vi "REMOND Studio_DO Water Q.vi"() -> ()   [LabVIEW 2021]
uses:
  FSM_States.ctl
  Global_Message.ctl
  <vilib>/Modbus/master/Modbus Master.lvclass
  <vilib>/Utility/error.llb/DialogType.ctl
  Global_flags.vi
  <vilib>/Modbus/master/Create Master Instance (Serial).vi
panel:
  in  "Measure Mode":u16(ring)=1 items=["[%]", "[mg/L]"]
  out "Tiempo Actual":string
  out "ADC":u16
  in  "Confirm Slope":bool
  in  "Confirm Zero":bool
  in  "Start Calib":bool
  out "Warning :":string
  out "Current Out Val :":sgl format="%#.3f"
  out "Temperature [°C]:":sgl format="%#.1f °C"
  out "Measurement [%  ; mg/L]:":sgl format="%#.2f mg/L"
  in  "Exit":bool
  in  "Restore Default":bool
  in  "Adquire / Stop":bool
  in  "SetBaudRate":bool
  in  "BaudRate (9600)":u16(ring)=2 items=["2400", "4800", "9600", "19200", "38400"]
  in  "Addr Set":u16=1 min=1 max=255 step=1
  in  "SetAddress":bool
  in  "D.S":u16(ring)=1 items=["0.5s", "1s", "1.5s", "2.0s", "2.5s", "3.0s", "3.5s", "4.0s", "4.5s", "5.0s"]
  in  "BaudRate (9600)":u32=9600 min=2400 max=38400 step=1
  in  "Address":u8=1 min=1 step=1
  in  "Open/Close COM":bool
  in  "COM":refnum<visa-resource-name>
  out "Consumer Shutdown?":bool
  # "Calibracion:"
  # "ADC :"
  # "Start CALIB --- >>> STOP ADQRUIING , DISble and gray out Measur and SHow ADC"
  # "Evento de filtrado Calib Slope Optional !!"
  # "Disable and gray out Measurements (Prop Node) while calibrating"
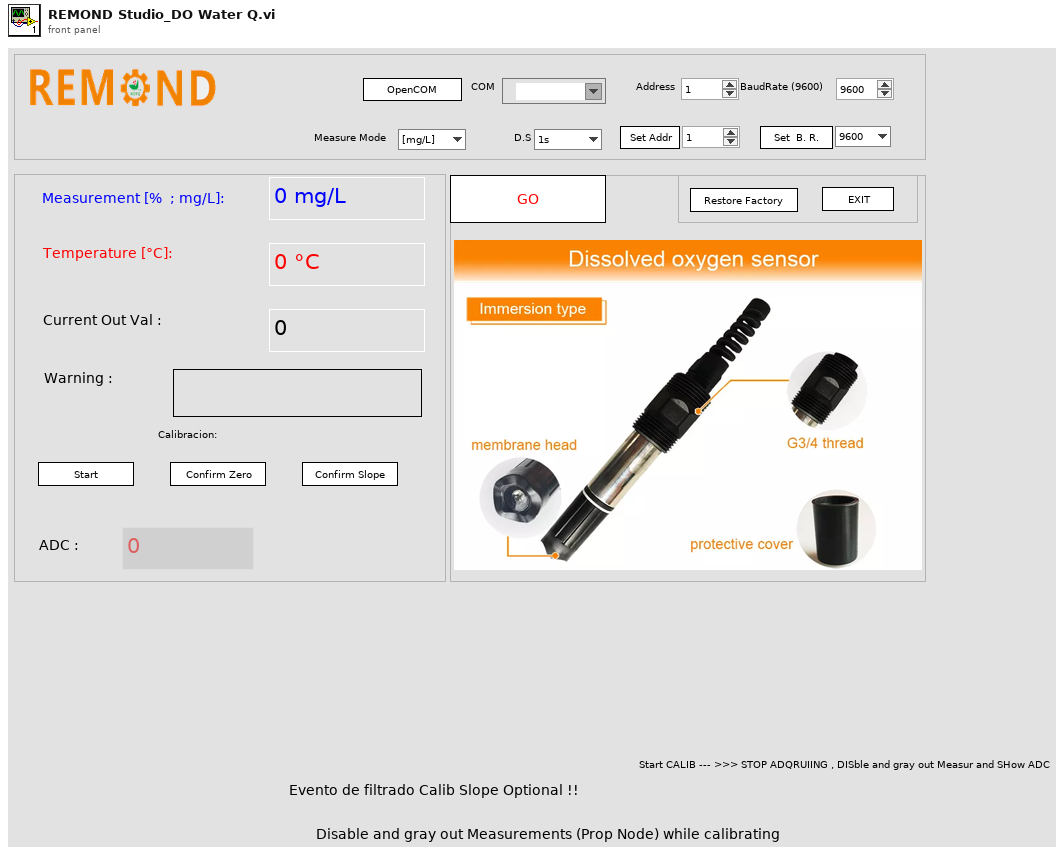
[diagram p1: front panel]
types:
  T1 = typedef "Global_Message.ctl" = cluster{"Consumer State":T2, "User Msg":string, "error in (no error)":errorcluster, "User Msg 2":string}
  T2 = typedef "FSM_States.ctl" = enum16{"Set Measure Mode", "Initialize", "Open COM Port", "Adquire Data", "Set Address", "Set BaudRate", "Restore Factory", "Pre-Set Zero", "Pre-Set K=1", "Pre-Set Slope", "Confirm Zero", "Confirm Slope", "Confirm EC", "Close COM Port", "Exit App", "Stop Data", "Calibrate sensor"}
  T3 = enum8{"Enabled", "Disabled", "Disabled and Grayed Out"}
  T4 = typedef "DialogType.ctl" = u16
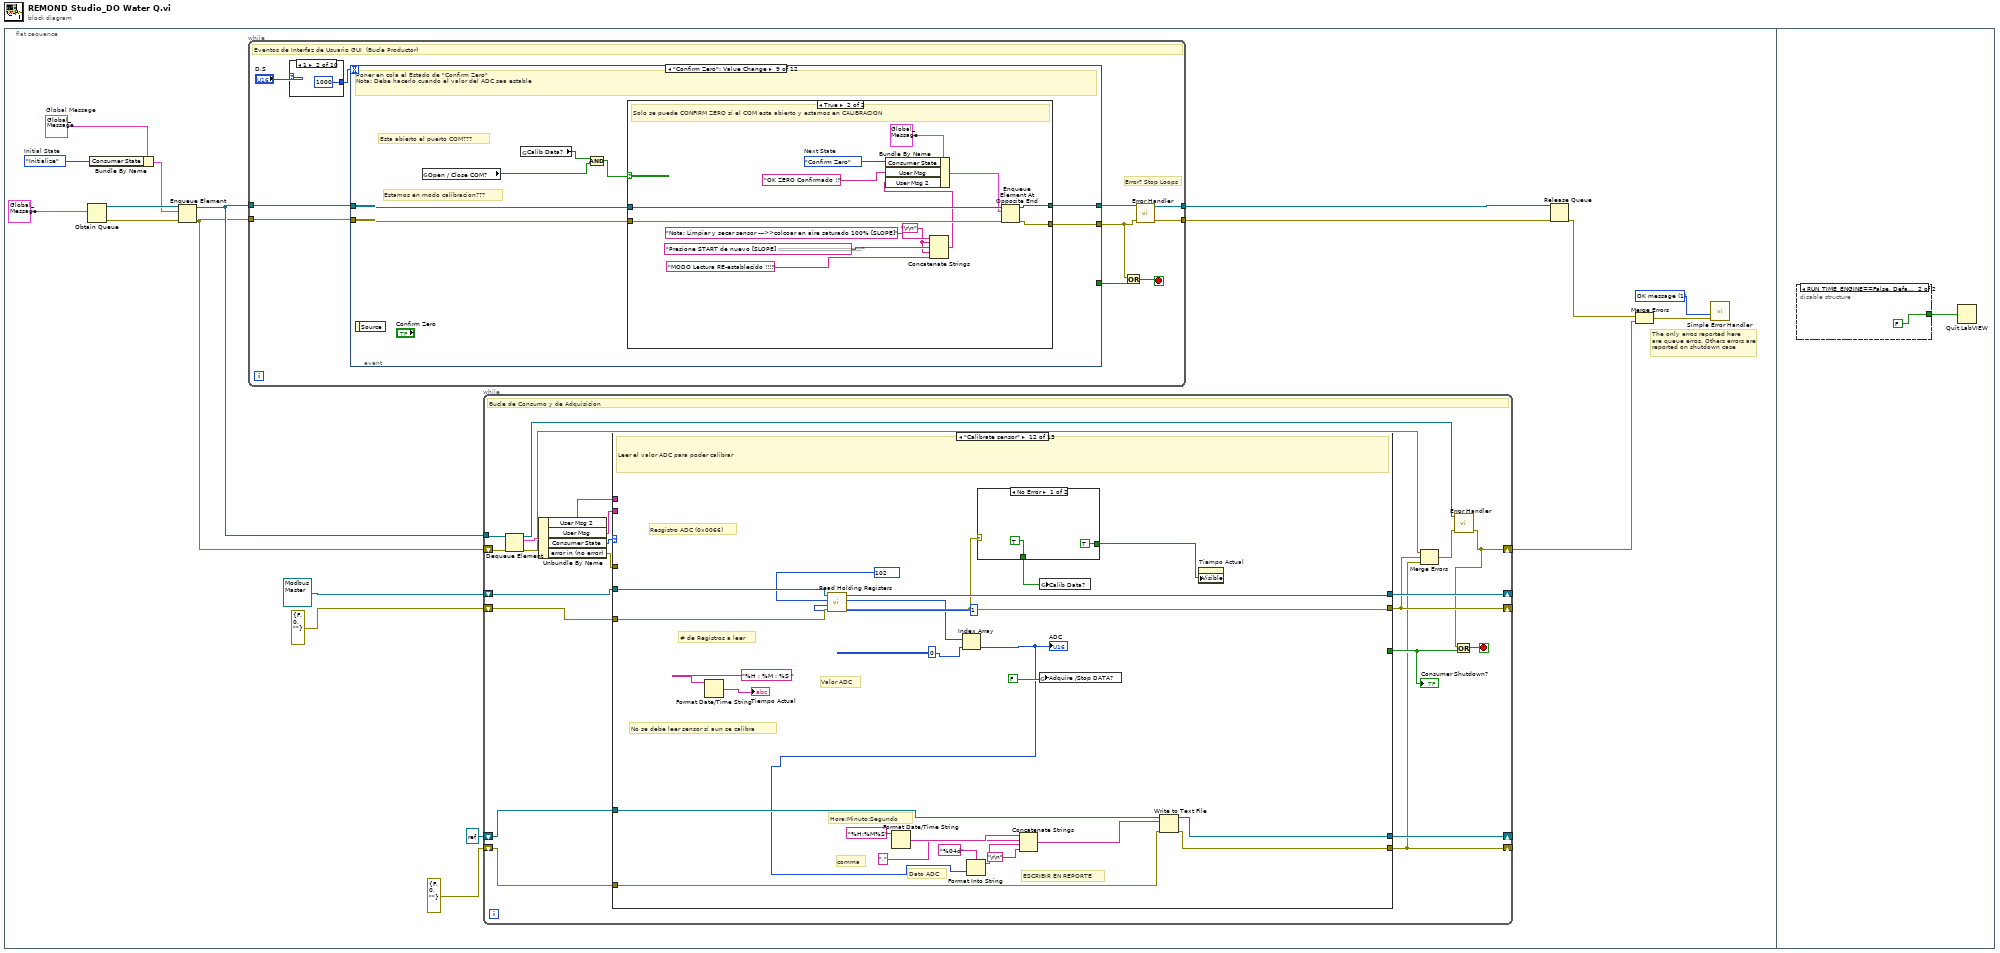
[diagram p0: block diagram]
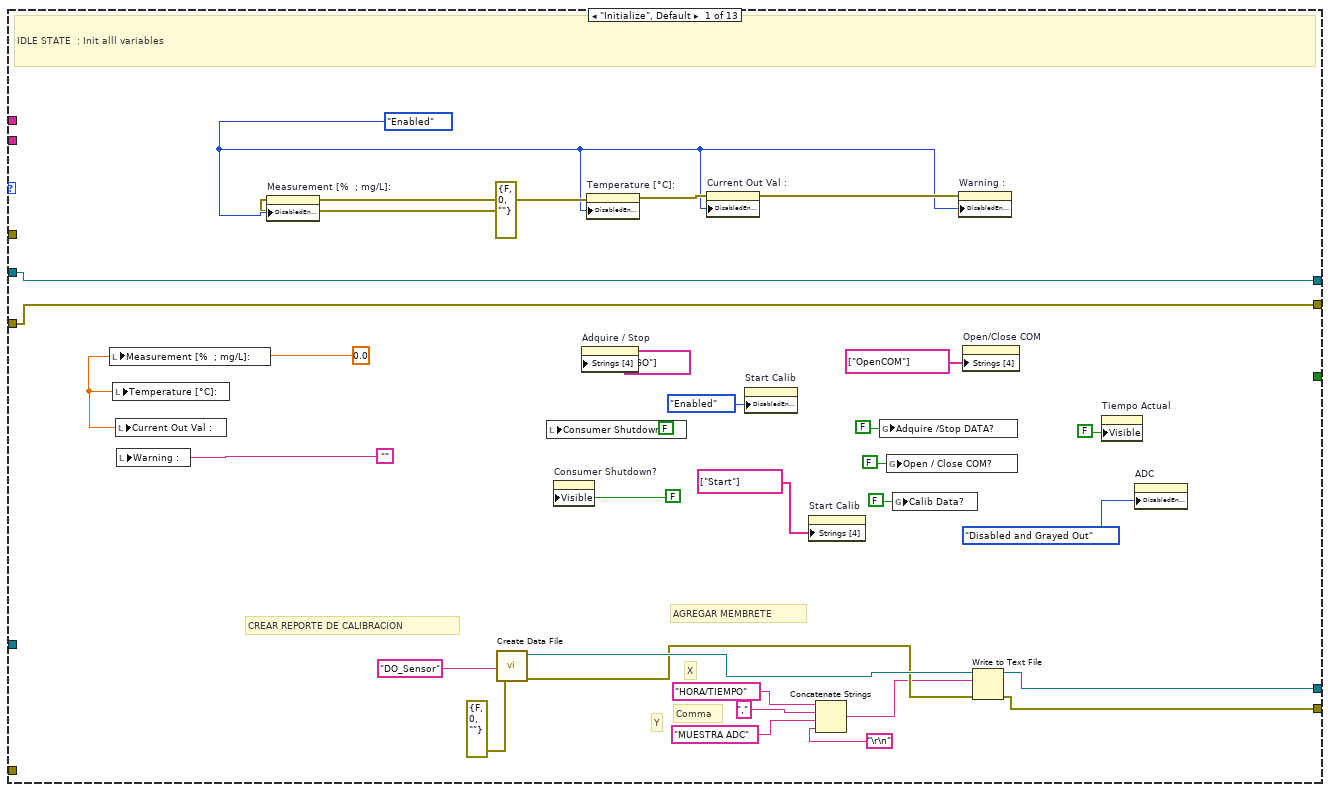
[diagram p2: hidden frame]
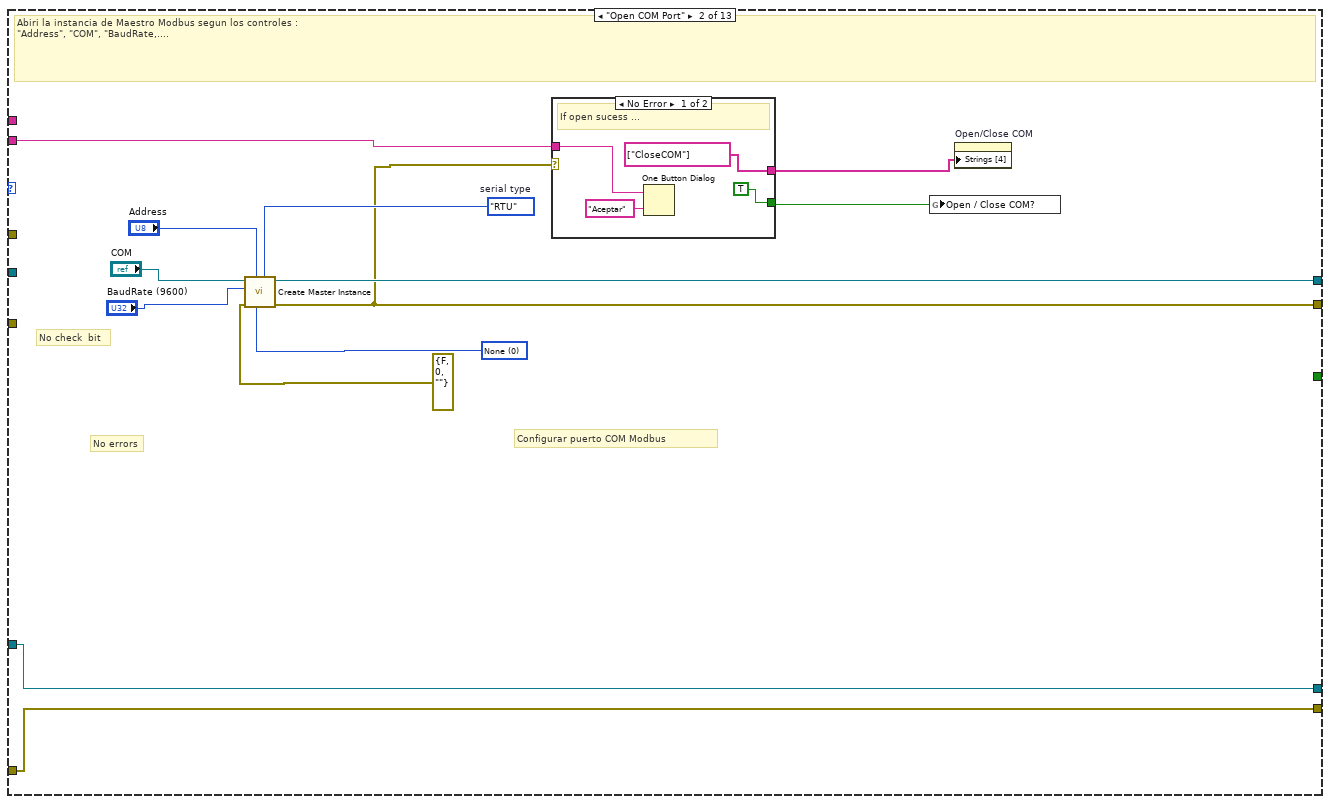
[diagram p3: hidden frame]
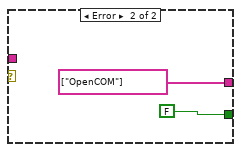
[diagram p4: hidden frame]
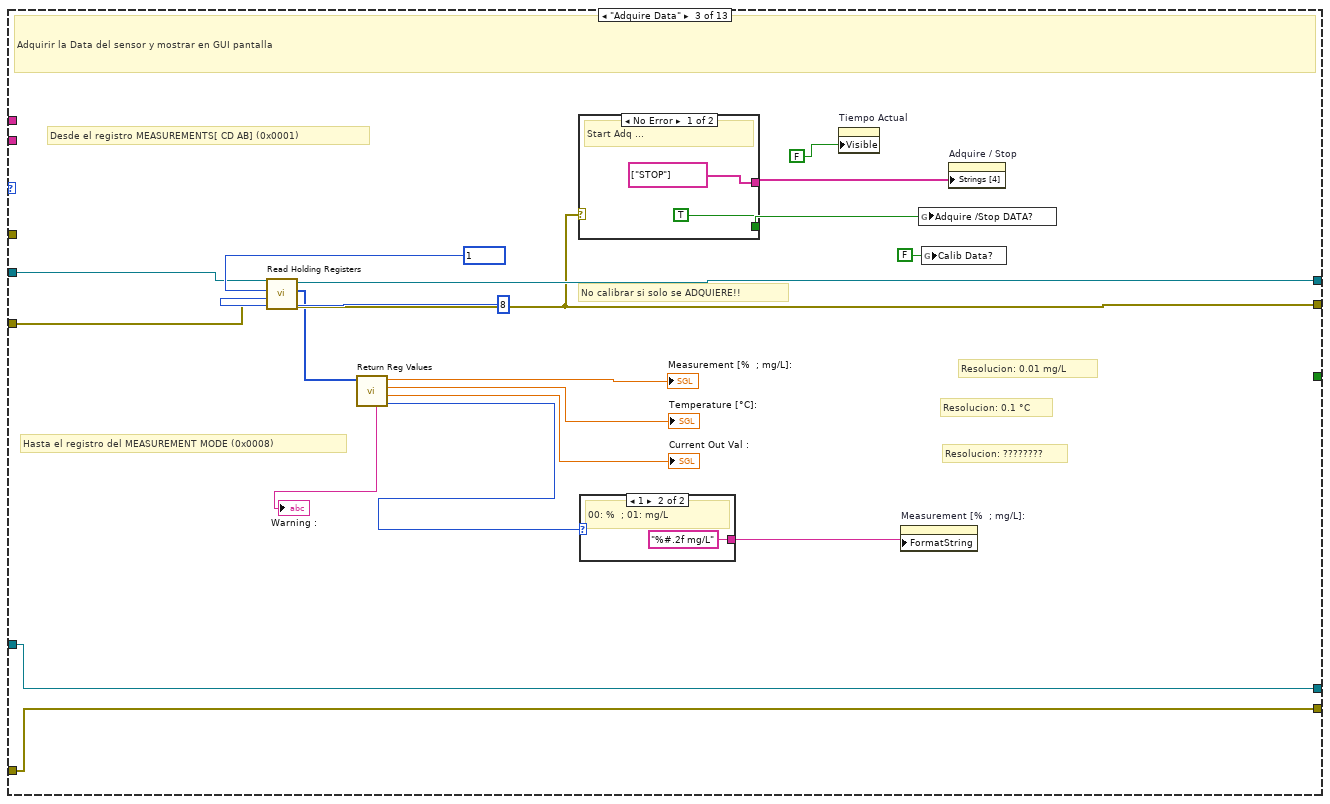
[diagram p5: hidden frame]
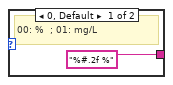
[diagram p6: hidden frame]
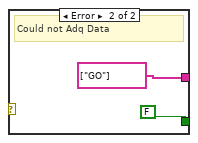
[diagram p7: hidden frame]
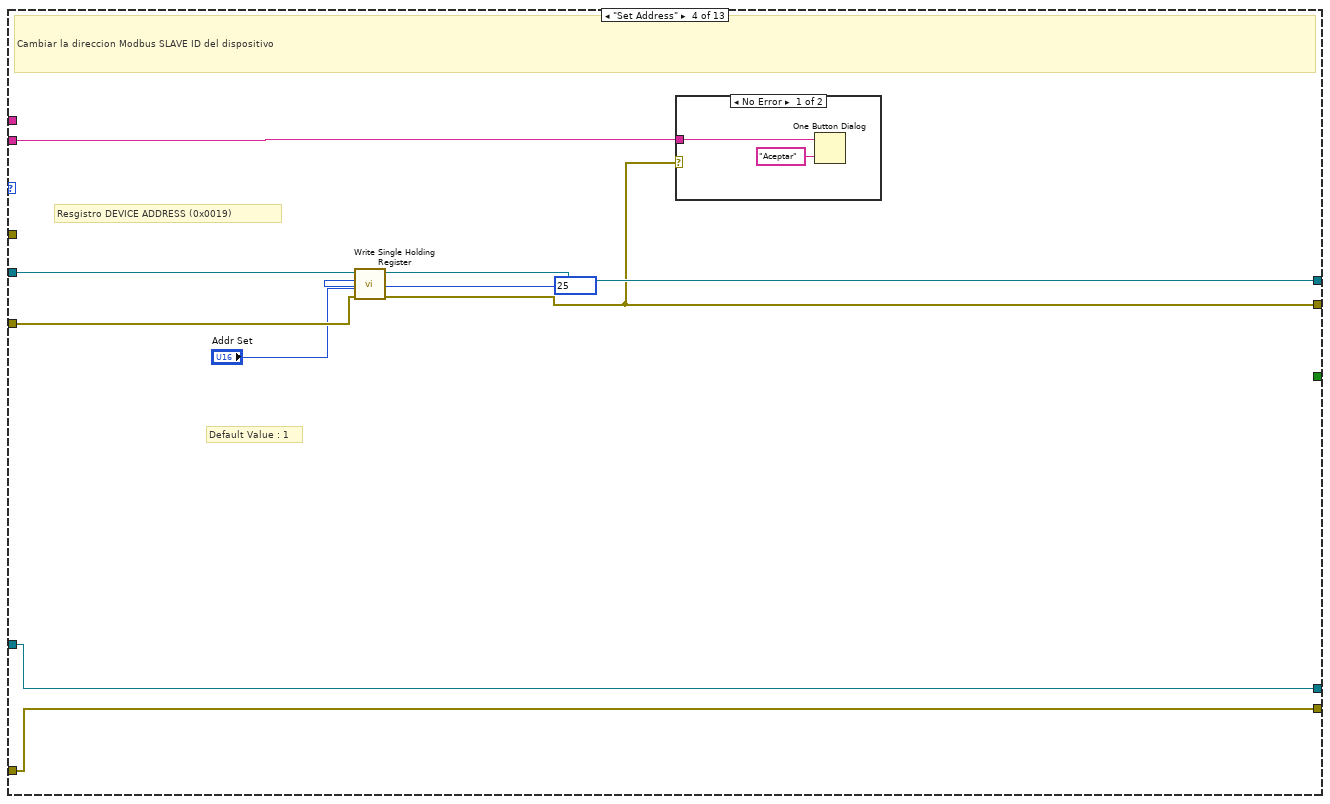
[diagram p8: hidden frame]
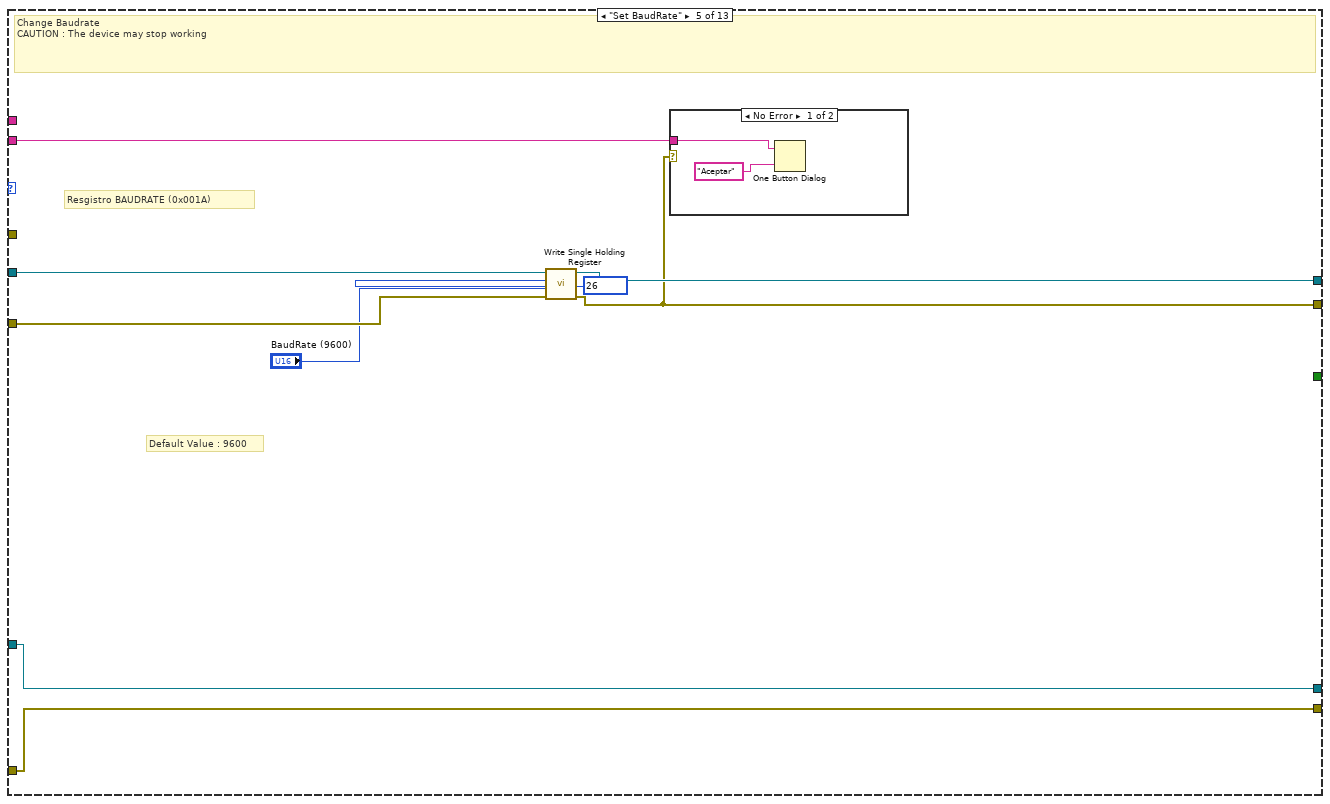
[diagram p10: hidden frame]
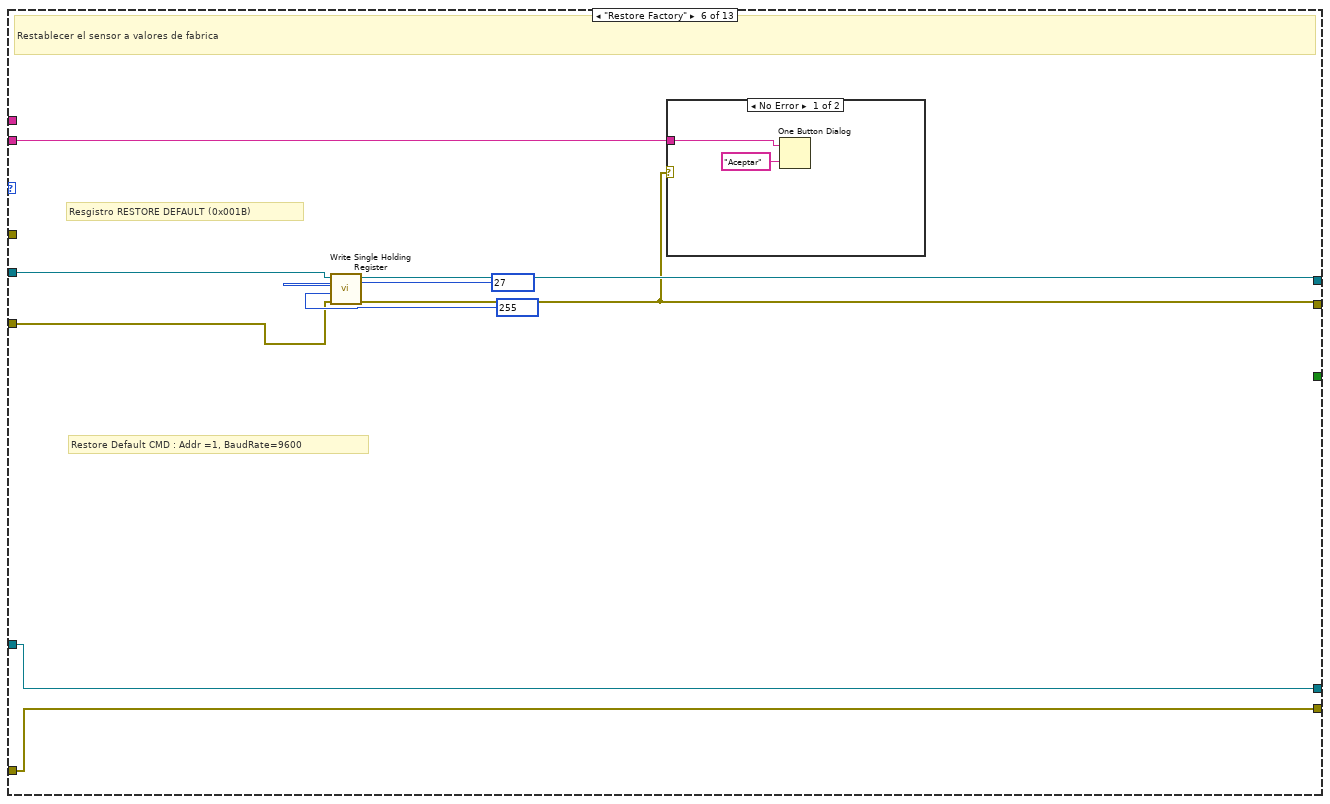
[diagram p12: hidden frame]
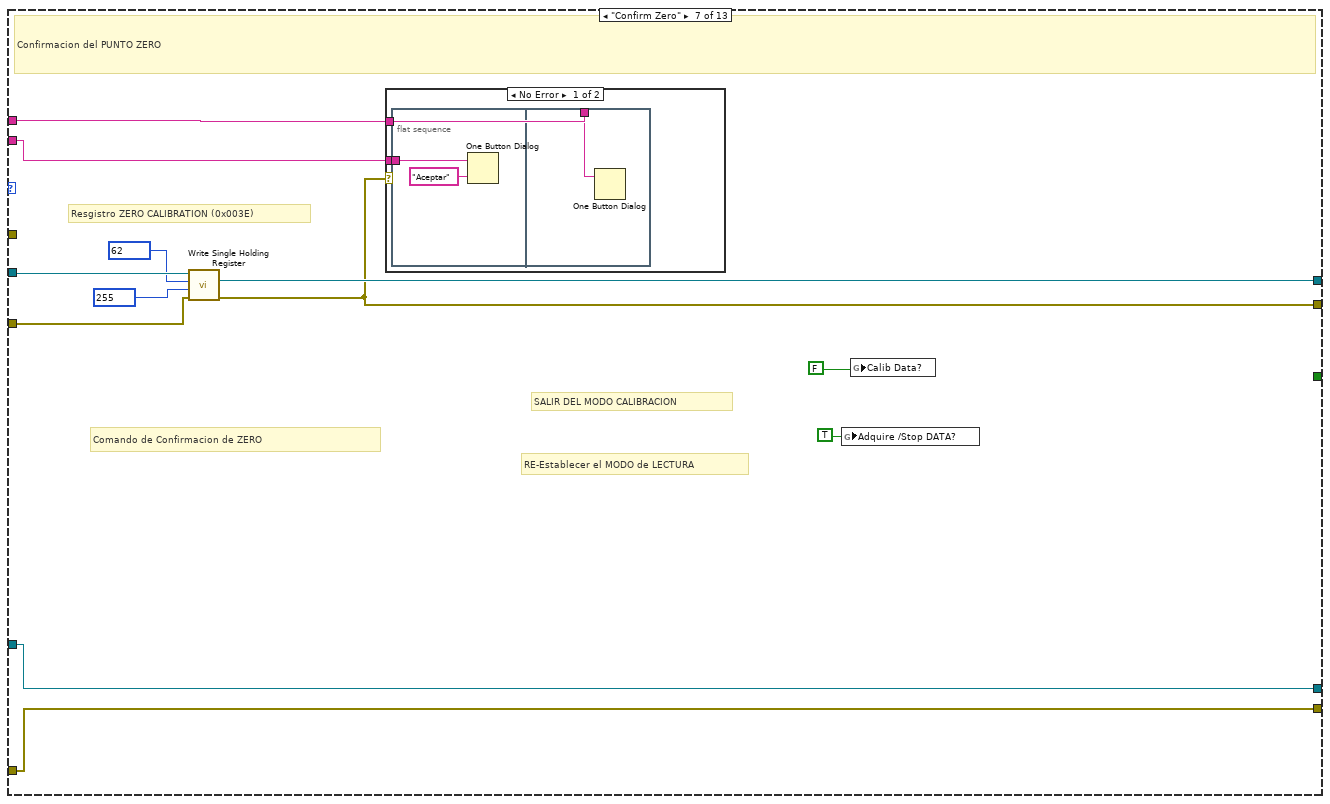
[diagram p14: hidden frame]
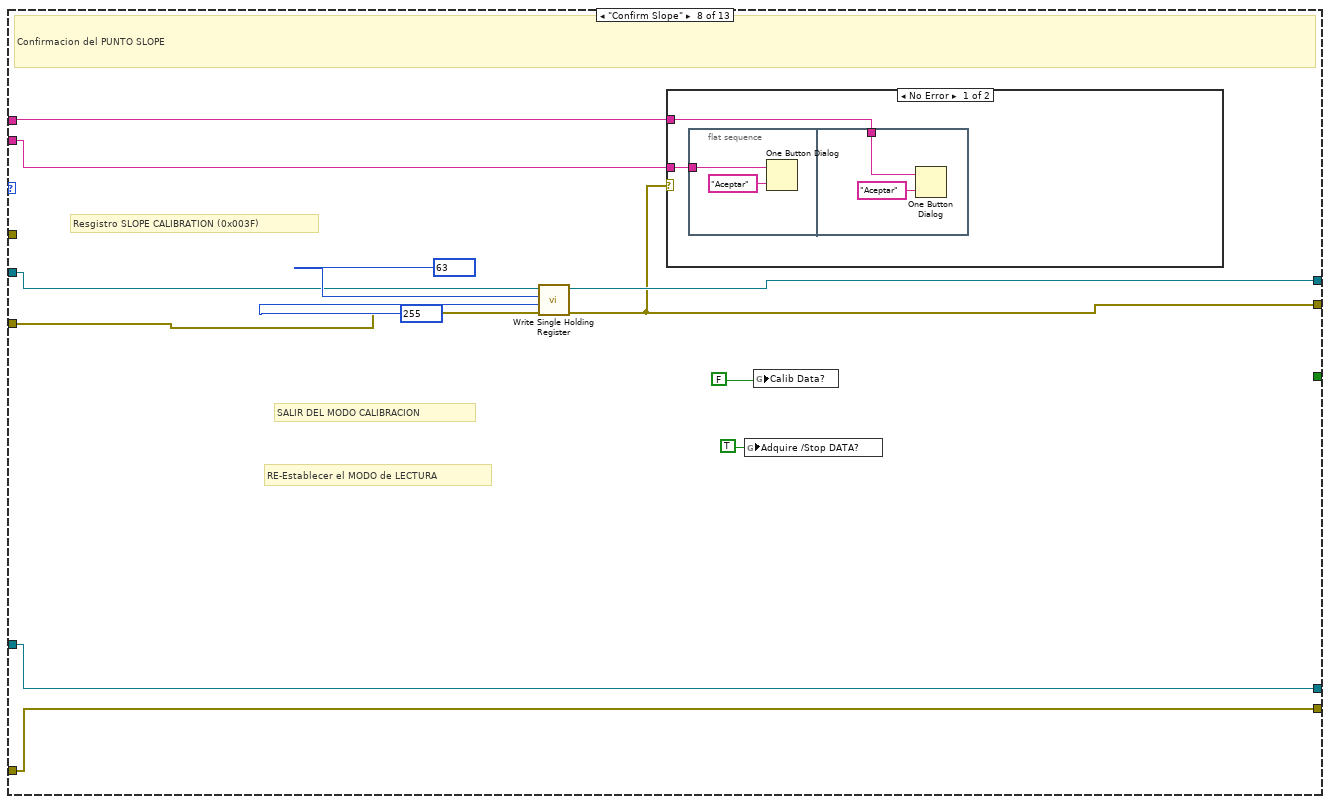
[diagram p16: hidden frame]
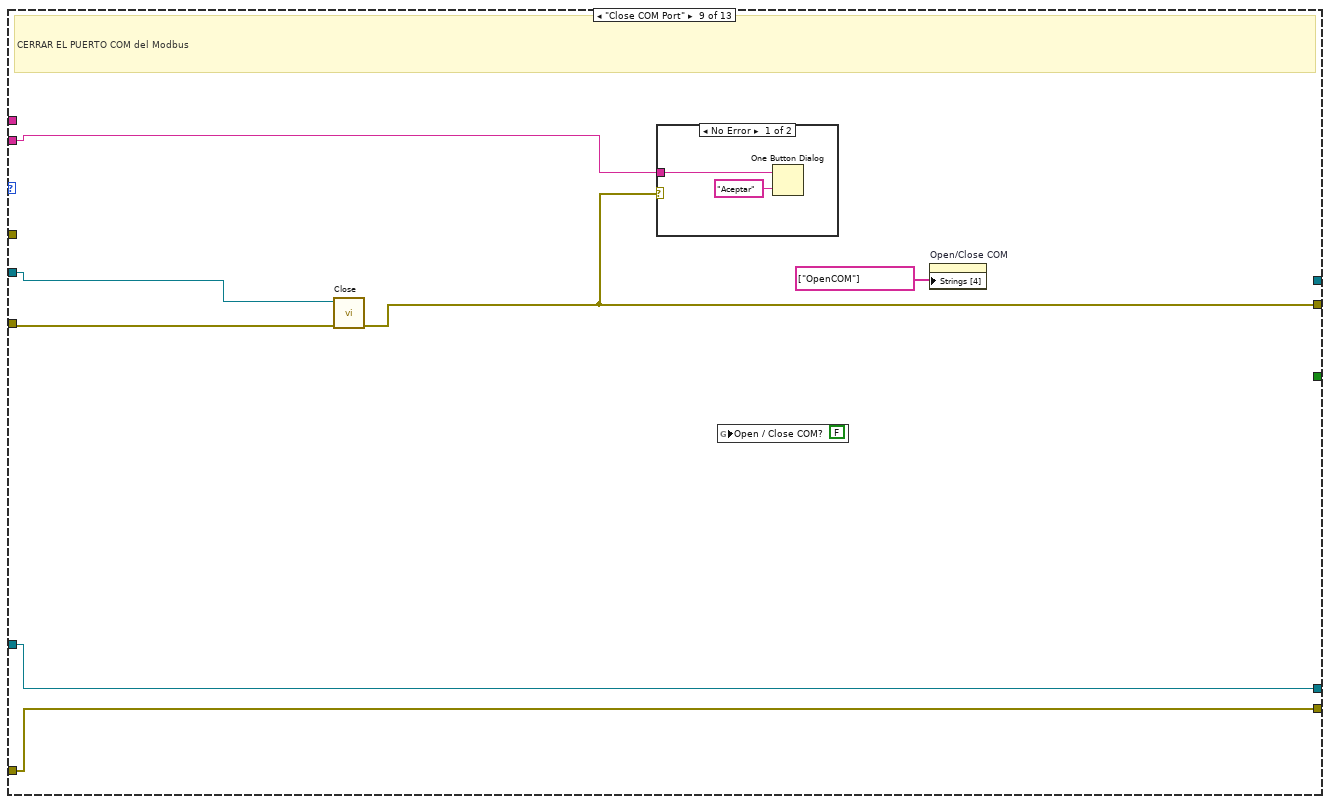
[diagram p18: hidden frame]
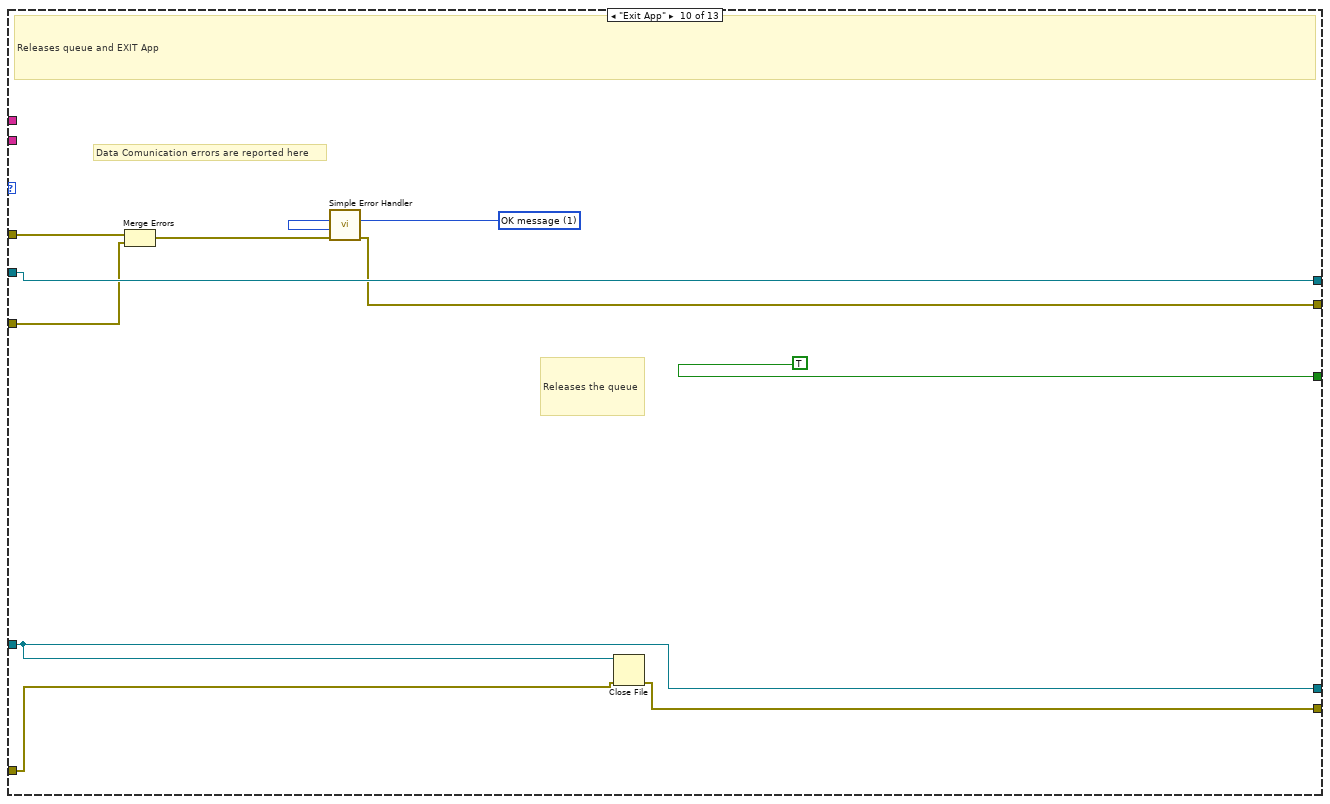
[diagram p20: hidden frame]
diagram:
  n1 = flat-sequence {
    frame #0 {
      w5 = T4 1 items=["no dialog", "OK message", "continue or stop message", "OK message + warnings", "continue/stop + warnings"] ("type of dialog (OK msg:1)")
      w15 = T1 {"Consumer State"=enum."Open COM Port", "User Msg"="", "error in (no error)"={"status"=FALSE, "code"=0, "source"=""}, "User Msg 2"=""}  # Global Message
      w14 = FSM_States."Initialize"  # Initial State
      # "The only erros reported here\nare queue erros. Others errors are\nreported on shutdown case"
      n2 = Obtain Queue(element data type=T1 {"Consumer State"=enum."Open COM Port", "User Msg"="", "error in (no error)"={"status"=FALSE, "code"=0, "source"=""}, "User Msg 2"=""} ("Global Message")) -> (queue out=w17:refnum<queue>, error out=w16:errorcluster)  [unwired: 4 in, 1 out]
      n3 = Bundle By Name(cluster=w15, "Consumer State"=w14) -> (w13:T1)
      n4 = Enqueue Element(queue=w17, element=w13, error in (no error)=w16) -> (queue out=w12:refnum<queue>, error out=w11:errorcluster)  [unwired: 1 in, 1 out]
      n5 = while {
        tunnel: w12 -> [w264]
        tunnel: w11 -> [w263]
        tunnel: [w259] -> w8
        tunnel: [w258] -> w7
        stop <- w255 stop-if-true
        # "Error? Stop Loops"
        # "Eventos de Interfaz de Usuario GUI  (Bucle Productor)"
        n6 = case shown="1" "D.S" {
          tunnel: [500 1000 1500 2000 2500 3000 3500 4000 4500 5000] -> w262
          frame 0, Default {
          }
          frame 1 {
          }
          frame 2 {
          }
          frame 3 {
          }
          frame 4 {
          }
          frame 5 {
          }
          frame 6 {
          }
          frame 7 {
          }
          frame 8 {
          }
          frame 9 {
          }
        }
        n7 = event shown="[8] \"Confirm Zero\": Value Change" {
          selector: _ -> [_ _ _ _ _ _ _ _ _ _ _ _]
          dyn-events: _ -> [_ _ _ _ _ _ _ _ _ _ _ _]
          timeout: w262 -> [_ _ _ _ _ _ _ _ _ _ _ _]
          tunnel: w264 -> [w285 w307 w322 w346 w383 w403 w423 w443 w485 w512 w537 w555]
          tunnel: w263 -> [w284 w306 w321 w345 w381 w401 w421 w441 w483 w510 w535 w554]
          tunnel: [w283 w305 w320 w344 w382 w402 w422 w442 w484 w511 w536 w555] -> w260
          tunnel: [w282 w304 w319 w343 w380 w400 w420 w440 w482 w509 w534 w554] -> w256
          tunnel: [w281 _ _ _ _ _ _ _ _ _ w532 _] -> w257
          event Timeout {
            # "Para ADQUIRIR DATOS, se debe ABRIR el PUERTO COM"
            # "Poner en cola el estado de \"ADQUIRE DATA\" de forma automatica cada 1000 mseg\n\nNOTA: Solo funcionara si el puerto COM esta abierto"
            n8 = event-data() -> ()  [unwired: 1 in, 1 out]
            n9 = global read "Global_flags.vi" "Adquire /Stop DATA?"() -> (w275:bool)
            n10 = case shown="True" w275 {
              frame False {
              }
              frame True {
                w286 = T3."Enabled" ("Disabled")
                # "Si se vuelve a adquirir, mostrar los controles"
                n11 = property on="Measurement [%  ; mg/L]:" class="DigNum (strict)"("DisabledEnum"=w286) -> ()  [unwired: 2 in, 2 out]
                n12 = property on="Temperature [°C]:" class="DigNum (strict)"("DisabledEnum"=w286) -> ()  [unwired: 2 in, 2 out]
                n13 = property on="Current Out Val :" class="DigNum (strict)"("DisabledEnum"=w286) -> ()  [unwired: 2 in, 2 out]
                n14 = property on="ADC" class="DigNum (strict)"("DisabledEnum"=T3."Disabled and Grayed Out" ("Disabled")) -> ()  [unwired: 2 in, 2 out]
                n15 = property on="Warning :" class="Str"("DisabledEnum"=w286) -> ()  [unwired: 2 in, 2 out]
                n16 = property on="Start Calib" class="Bool"("DisabledEnum"=w286) -> ()  [unwired: 2 in, 2 out]
              }
            }
            n17 = global read "Global_flags.vi" "Calib Data?"() -> (w280:bool)
            n18 = global read "Global_flags.vi" "Open / Close COM?"() -> (w278:bool)
            n19 = Build Array(w275, w280) -> (w279:bool[])
            n20 = And(x=w279, y=w278) -> (x .and. y?=w277:bool[])
            n21 = Boolean Array To Number(Boolean array=w277) -> (number=w276:u32)
            n22 = case shown="2" w276 {
              tunnel: [w289 w294 w300] -> w283
              tunnel: [w288 w293 w298] -> w282
              tunnel: w285 -> [w289 w291 w301]
              tunnel: w284 -> [w288 w290 w299]
              frame 0, Default {
                # "Caso contrario, Bypass"
              }
              frame 1 {
                w292 = FSM_States."Adquire Data"  # Next State
                # "Si Adq/Stop ==True entonces ADQUIRIR"
                n23 = Bundle By Name(cluster=T1 {"Consumer State"=enum."Open COM Port", "User Msg"="", "error in (no error)"={"status"=FALSE, "code"=0, "source"=""}, "User Msg 2"=""} ("Global Message"), "Consumer State"=w292) -> (w295:T1)
                n24 = Enqueue Element(queue=w291, element=w295, error in (no error)=w290) -> (queue out=w294:refnum<queue>, error out=w293:errorcluster)  [unwired: 1 in, 1 out]
              }
              frame 2 {
                w303 = FSM_States."Calibrate sensor"  # Next State
                # "Si Calib Data? == True entonces calibrar sensor"
                n25 = Bundle By Name(cluster=T1 {"Consumer State"=enum."Open COM Port", "User Msg"="", "error in (no error)"={"status"=FALSE, "code"=0, "source"=""}, "User Msg 2"=""} ("Global Message"), "Consumer State"=w303) -> (w297:T1)
                n26 = Enqueue Element(queue=w301, element=w297, error in (no error)=w299) -> (queue out=w300:refnum<queue>, error out=w298:errorcluster)  [unwired: 1 in, 1 out]
              }
            }
            n27 = local read "Consumer Shutdown?"() -> (w281:bool)
          }
          event "Open/Close COM": Value Change {
            w313 = FSM_States."Close COM Port"  # Next State
            w314 = FSM_States."Open COM Port"  # Next State
            # "Poner en cola en estado de apertura de puerto COM Modbus"
            n28 = event-data() -> ()  [unwired: 1 in, 1 out]
            n29 = global read "Global_flags.vi" "Open / Close COM?"() -> (w311:bool)
            n30 = Select(t="Puerto COM cerrado !", s=w311, f="Puerto COM abierto !" ("User Msg")) -> (s? t:f=w310:string)
            n31 = Select(t=w313, s=w311, f=w314) -> (s? t:f=w316:T2)
            n32 = Bundle By Name(cluster=T1 {"Consumer State"=enum."Open COM Port", "User Msg"="", "error in (no error)"={"status"=FALSE, "code"=0, "source"=""}, "User Msg 2"=""} ("Global Message"), "Consumer State"=w316, "User Msg"=w310) -> (w309:T1)
            n33 = Enqueue Element(queue=w307, element=w309, error in (no error)=w306) -> (queue out=w305:refnum<queue>, error out=w304:errorcluster)  [unwired: 1 in, 1 out]
          }
          event "Measure Mode": Value Change {
            # "Esta abierto el puerto COM???"
            # "Poner en cola en estado de MODO\nNOTA: Solo funcionara si el COM esta abierto"
            n34 = event-data() -> ()  [unwired: 1 in, 4 out]
            n35 = global read "Global_flags.vi" "Open / Close COM?"() -> (w318:bool)
            n36 = case shown="True" w318 {
              tunnel: w322 -> [w324 w335]
              tunnel: w321 -> [w323 w334]
              tunnel: [w324 w333] -> w320
              tunnel: [w323 w332] -> w319
              tunnel: "Measure Mode" -> [_ w331]
              frame False {
                # "Solo se puede SET MEASU MODE si el COM esta abierto"
                n37 = Concatenate Strings("Para cambiar MEASURE MODE::::::" ("message"), "\r\n", "Debe ABRIR Puerto COM !!!" ("string")) -> (w329:string)
                n38 = One Button Dialog(message=w329, button name ("OK")="Aceptar") -> ()  [unwired: 1 out]
              }
              frame True {
                w338 = FSM_States."Set Measure Mode"  # Next State
                # "Solo se puede SET MEASU MODE si el COM esta abierto"
                n39 = case shown="0, Default" w331 {
                  tunnel: ["%" "mg/L"] -> w330
                  frame 0, Default {
                  }
                  frame 1 {
                  }
                }
                n40 = Bundle By Name(cluster=T1 {"Consumer State"=enum."Open COM Port", "User Msg"="", "error in (no error)"={"status"=FALSE, "code"=0, "source"=""}, "User Msg 2"=""} ("Global Message"), "Consumer State"=w338, "User Msg"="OK Measure Mode Changed!!! !!", "User Msg 2"=w330) -> (w336:T1)
                n41 = Enqueue Element(queue=w335, element=w336, error in (no error)=w334) -> (queue out=w333:refnum<queue>, error out=w332:errorcluster)  [unwired: 1 in, 1 out]
              }
            }
          }
          event "Adquire / Stop": Value Change {
            # "Esta abierto el puerto COM???"
            # "Ya se esta adquiriendo???"
            # "Poner en cola en estado de adquisicion de muestras\nNOTA: Solo funcionara si el COM esta abierto"
            n42 = event-data() -> ()  [unwired: 1 in, 1 out]
            n43 = global read "Global_flags.vi" "Adquire /Stop DATA?"() -> (w347:bool)
            n44 = global read "Global_flags.vi" "Open / Close COM?"() -> (w342:bool)
            n45 = case shown="True" w342 {
              tunnel: w347 -> [_ w364]
              tunnel: w346 -> [w354 w363]
              tunnel: w345 -> [w353 w362]
              tunnel: [w354 w361] -> w344
              tunnel: [w353 w360] -> w343
              frame False {
                # "Solo se puede ADQUIRIR si el COM esta abierto"
                n46 = Concatenate Strings("Para ADQUIRI muestras::::::" ("message"), "\r\n", "Debe ABRIR Puerto COM !!!" ("string")) -> (w348:string)
                n47 = One Button Dialog(message=w348, button name ("OK")="Aceptar") -> ()  [unwired: 1 out]
              }
              frame True {
                w355 = T3."Enabled" ("Disabled")
                w356 = errorcluster {"status"=FALSE, "code"=0, "source"=""} ("error in (no error)")
                # "Solo se puede ADQUIRIR si el COM esta abierto"
                n48 = property on="Measurement [%  ; mg/L]:" class="DigNum (strict)"(error in=w356, "DisabledEnum"=w355) -> (error out=w359:errorcluster)  [unwired: 1 in, 1 out]
                n49 = property on="Start Calib" class="Bool"(error in=w356, "DisabledEnum"=w355) -> ()  [unwired: 1 in, 2 out]
                n50 = case shown="True" w364 {
                  tunnel: [w369 w375] -> w361
                  tunnel: [w368 w374] -> w360
                  tunnel: w363 -> [w366 w373]
                  tunnel: w362 -> [w365 w372]
                  frame False {
                    w367 = FSM_States."Adquire Data"  # Next State
                    # "Si no se ha iniciado la adquisicion  encolar ADQUIRIR"
                    n51 = Bundle By Name(cluster=T1 {"Consumer State"=enum."Open COM Port", "User Msg"="", "error in (no error)"={"status"=FALSE, "code"=0, "source"=""}, "User Msg 2"=""} ("Global Message"), "Consumer State"=w367) -> (w370:T1)
                    n52 = Enqueue Element(queue=w366, element=w370, error in (no error)=w365) -> (queue out=w369:refnum<queue>, error out=w368:errorcluster)  [unwired: 1 in, 1 out]
                  }
                  frame True {
                    w376 = FSM_States."Stop Data"  # Next State
                    # "Si ya se estaba adquiriendo, DETENER la toma de data"
                    n53 = Bundle By Name(cluster=T1 {"Consumer State"=enum."Open COM Port", "User Msg"="", "error in (no error)"={"status"=FALSE, "code"=0, "source"=""}, "User Msg 2"=""} ("Global Message"), "Consumer State"=w376) -> (w377:T1)
                    n54 = Enqueue Element(queue=w373, element=w377, error in (no error)=w372) -> (queue out=w375:refnum<queue>, error out=w374:errorcluster)  [unwired: 1 in, 1 out]
                  }
                }
                n55 = property on="Temperature [°C]:" class="DigNum (strict)"(error in=w359, "DisabledEnum"=w355) -> (error out=w358:errorcluster)  [unwired: 1 in, 1 out]
                n56 = property on="Current Out Val :" class="DigNum (strict)"(error in=w358, "DisabledEnum"=w355) -> (error out=w357:errorcluster)  [unwired: 1 in, 1 out]
                n57 = property on="Warning :" class="Str"(error in=w357, "DisabledEnum"=w355) -> ()  [unwired: 1 in, 2 out]
              }
            }
          }
          event "SetAddress": Value Change {
            # "Esta abierto el puerto COM???"
            # "Poner en cola el Estado de Set Address\nNOTA: Solo funcionara si el COM esta abierto"
            n58 = event-data() -> ()  [unwired: 1 in, 1 out]
            n59 = global read "Global_flags.vi" "Open / Close COM?"() -> (w379:bool)
            n60 = case shown="False" w379 {
              tunnel: w383 -> [w390 w396]
              tunnel: [w390 w395] -> w382
              tunnel: w381 -> [w389 w394]
              tunnel: [w389 w393] -> w380
              frame False {
                # "Solo se puede SetAddr si el COM esta abierto"
                n61 = Concatenate Strings("Para cambiar SLAVE ID::::::" ("message"), "\r\n", "Debe ABRIR Puerto COM !!!" ("string")) -> (w388:string)
                n62 = One Button Dialog(message=w388, button name ("OK")="Aceptar") -> ()  [unwired: 1 out]
              }
              frame True {
                w397 = FSM_States."Set Address"  # Next State
                # "Solo se puede SET ADDR si el COM esta abierto"
                n63 = Bundle By Name(cluster=T1 {"Consumer State"=enum."Open COM Port", "User Msg"="", "error in (no error)"={"status"=FALSE, "code"=0, "source"=""}, "User Msg 2"=""} ("Global Message"), "Consumer State"=w397, "User Msg"="OK Set Address !!") -> (w392:T1)
                n64 = Enqueue Element(queue=w396, element=w392, error in (no error)=w394) -> (queue out=w395:refnum<queue>, error out=w393:errorcluster)  [unwired: 1 in, 1 out]
              }
            }
          }
          event "SetBaudRate": Value Change {
            # "Esta abierto el puerto COM???"
            # "Poner en cola el Estado de Set Baudrate: Modifica el Baudrate\nNota: Solo funcionara si el COM esta abierto"
            n65 = event-data() -> ()  [unwired: 1 in, 1 out]
            n66 = global read "Global_flags.vi" "Open / Close COM?"() -> (w399:bool)
            n67 = case shown="True" w399 {
              tunnel: w403 -> [w405 w416]
              tunnel: [w405 w415] -> w402
              tunnel: w401 -> [w404 w414]
              tunnel: [w404 w413] -> w400
              frame False {
                # "Solo se puede SetBAUD si el COM esta abierto"
                n68 = Concatenate Strings("Para cambiar BAUDRATE::::::" ("message"), "\r\n", "Debe ABRIR Puerto COM !!!" ("string")) -> (w410:string)
                n69 = One Button Dialog(message=w410, button name ("OK")="Aceptar") -> ()  [unwired: 1 out]
              }
              frame True {
                w417 = FSM_States."Set BaudRate"  # Next State
                # "Solo se puede SetBAUD si el COM esta abierto"
                n70 = Bundle By Name(cluster=T1 {"Consumer State"=enum."Open COM Port", "User Msg"="", "error in (no error)"={"status"=FALSE, "code"=0, "source"=""}, "User Msg 2"=""} ("Global Message"), "Consumer State"=w417, "User Msg"="OK Set BaudRate !!") -> (w412:T1)
                n71 = Enqueue Element(queue=w416, element=w412, error in (no error)=w414) -> (queue out=w415:refnum<queue>, error out=w413:errorcluster)  [unwired: 1 in, 1 out]
              }
            }
          }
          event "Restore Default": Value Change {
            # "Esta abierto el puerto COM???"
            # "Poner en cola el Estado de Set Baudrate: Modifica el Baudrate\nNota: Solo funcionara si el COM esta abierto"
            n72 = event-data() -> ()  [unwired: 1 in, 1 out]
            n73 = global read "Global_flags.vi" "Open / Close COM?"() -> (w419:bool)
            n74 = case shown="True" w419 {
              tunnel: w423 -> [w430 w435]
              tunnel: [w430 w434] -> w422
              tunnel: w421 -> [w429 w433]
              tunnel: [w429 w432] -> w420
              frame False {
                # "Solo se puede RESTDEFAULT si el COM esta abierto"
                n75 = Concatenate Strings("Para RESTORE DEFAULT::::::" ("message"), "\r\n", "Debe ABRIR Puerto COM !!!" ("string")) -> (w428:string)
                n76 = One Button Dialog(message=w428, button name ("OK")="Aceptar") -> ()  [unwired: 1 out]
              }
              frame True {
                w437 = FSM_States."Restore Factory"  # Next State
                # "Solo se puede RESTDEFAULT si el COM esta abierto"
                n77 = Bundle By Name(cluster=T1 {"Consumer State"=enum."Open COM Port", "User Msg"="", "error in (no error)"={"status"=FALSE, "code"=0, "source"=""}, "User Msg 2"=""} ("Global Message"), "Consumer State"=w437, "User Msg"="OK Restore Factory !!") -> (w431:T1)
                n78 = Enqueue Element(queue=w435, element=w431, error in (no error)=w433) -> (queue out=w434:refnum<queue>, error out=w432:errorcluster)  [unwired: 1 in, 1 out]
              }
            }
          }
          event "Start Calib": Value Change {
            # "Esta abierto el puerto COM???"
            # "Poner en cola en Estado de \"Start Calibration\""
            n79 = event-data() -> ()  [unwired: 1 in, 1 out]
            n80 = global read "Global_flags.vi" "Open / Close COM?"() -> (w439:bool)
            n81 = case shown="True" w439 {
              tunnel: w443 -> [w450 w463]
              tunnel: [w450 w462] -> w442
              tunnel: w441 -> [w449 w461]
              tunnel: [w449 w460] -> w440
              frame False {
                # "Solo se puede START CALIB si el COM esta abierto"
                n82 = Concatenate Strings("Para EMPEZAR CALIBRACION::::::" ("message"), "\r\n", "Debe ABRIR Puerto COM !!!" ("string")) -> (w448:string)
                n83 = One Button Dialog(message=w448, button name ("OK")="Aceptar") -> ()  [unwired: 1 out]
              }
              frame True {
                w452 = T3."Disabled and Grayed Out" ("Disabled")
                # "Solo se puede START CALIB si el COM esta abierto"
                n84 = flat-sequence {
                  tunnel: w461 -> [w470]
                  tunnel: w463 -> [w471]
                  tunnel: [w471] -> w459
                  tunnel: [w470] -> w458
                  tunnel: [w475] -> w462
                  tunnel: [w473] -> w460
                  tunnel: w459 -> [w476]
                  tunnel: w458 -> [w474]
                  frame #0 {
                    w465 = "\r\n"
                    n85 = Concatenate Strings("Modo de calibracion INCIADO! " ("string"), w465, "NOTA: Sumerga el sensor en Sol. Estand [Sodium Sulfite 0% D0] o aire saturado al 100% " ("string"), w465, w465, "Presione \"Confirm Zero\" o \"Confirm Slope\" segun el caso " ("string")) -> (w467:string)
                    n86 = One Button Dialog(message=w467, button name ("OK")="Aceptar") -> ()  [unwired: 1 out]
                  }
                  frame #1 {
                    w477 = FSM_States."Calibrate sensor"  # Next State
                    n87 = Bundle By Name(cluster=T1 {"Consumer State"=enum."Open COM Port", "User Msg"="", "error in (no error)"={"status"=FALSE, "code"=0, "source"=""}, "User Msg 2"=""} ("Global Message"), "Consumer State"=w477) -> (w472:T1)
                    n88 = Enqueue Element(queue=w476, element=w472, error in (no error)=w474) -> (queue out=w475:refnum<queue>, error out=w473:errorcluster)  [unwired: 1 in, 1 out]
                  }
                }
                n89 = property on="ADC" class="DigNum (strict)"("DisabledEnum"=T3."Enabled" ("Disabled")) -> ()  [unwired: 2 in, 2 out]
                n90 = property on="Measurement [%  ; mg/L]:" class="DigNum (strict)"(error in=errorcluster {"status"=FALSE, "code"=0, "source"=""} ("error in (no error)"), "DisabledEnum"=w452) -> (error out=w455:errorcluster)  [unwired: 1 in, 1 out]
                n91 = property on="Temperature [°C]:" class="DigNum (strict)"(error in=w455, "DisabledEnum"=w452) -> (error out=w456:errorcluster)  [unwired: 1 in, 1 out]
                n92 = property on="Current Out Val :" class="DigNum (strict)"(error in=w456, "DisabledEnum"=w452) -> (error out=w457:errorcluster)  [unwired: 1 in, 1 out]
                n93 = property on="Warning :" class="Str"(error in=w457, "DisabledEnum"=w452) -> (error out=w453:errorcluster)  [unwired: 1 in, 1 out]
                n94 = property on="Start Calib" class="Bool"(error in=w453, "DisabledEnum"=w452) -> ()  [unwired: 1 in, 2 out]
              }
            }
          }
          event "Confirm Zero": Value Change {
            # "Estamos en modo calibracion???"
            # "Esta abierto el puerto COM???"
            # "Poner en cola el Estado de \"Confirm Zero\"\nNota: Debe hacerlo cuando el valor del ADC sea estable"
            n95 = event-data() -> ()  [unwired: 1 in, 1 out]
            n96 = global read "Global_flags.vi" "Open / Close COM?"() -> (w479:bool)
            n97 = global read "Global_flags.vi" "Calib Data?"() -> (w481:bool)
            n98 = And(x=w481, y=w479) -> (x .and. y?=w480:bool)
            n99 = case shown="True" w480 {
              tunnel: w485 -> [w492 w503]
              tunnel: [w492 w502] -> w484
              tunnel: w483 -> [w491 w501]
              tunnel: [w491 w500] -> w482
              frame False {
                # "Solo se puede CONFIRM ZERO si el COM esta abierto y estamos en CALIBRACION"
                n100 = Concatenate Strings("Para CONFIRMAR ZERO::::::" ("message"), "\r\n", "Debe ABRIR Puerto COM o Start Calibracion (ADC) Primero !!!" ("string")) -> (w490:string)
                n101 = One Button Dialog(message=w490, button name ("OK")="Aceptar") -> ()  [unwired: 1 out]
              }
              frame True {
                w494 = "\r\n"
                w504 = FSM_States."Confirm Zero"  # Next State
                # "Solo se puede CONFIRM ZERO si el COM esta abierto y estamos en CALIBRACION"
                n102 = Concatenate Strings("Nota: Limpiar y secar sensor --->>colcoar en aire saturado 100% [SLOPE]" ("User Msg 2"), w494, "Presione START de nuevo [SLOPE] ::::::::::::::::::::::::::::::::::::::::::" ("string"), w494, "MODO Lectura RE-establecido !!!!" ("string")) -> (w496:string)
                n103 = Bundle By Name(cluster=T1 {"Consumer State"=enum."Open COM Port", "User Msg"="", "error in (no error)"={"status"=FALSE, "code"=0, "source"=""}, "User Msg 2"=""} ("Global Message"), "Consumer State"=w504, "User Msg"="OK ZERO Confirmado !!", "User Msg 2"=w496) -> (w499:T1)
                n104 = Enqueue Element At Opposite End(queue=w503, element=w499, error in (no error)=w501) -> (queue out=w502:refnum<queue>, error out=w500:errorcluster)  [unwired: 1 in, 1 out]
              }
            }
          }
          event "Confirm Slope": Value Change {
            # "Estamos en modo calibracion???"
            # "Esta abierto el puerto COM???"
            # "Poner en cola el Estado de \"Confirm Slope\"\nNota: Debe hacerlo cuando el valor del ADC sea estable y luego de haber confirmado el zero"
            n105 = event-data() -> ()  [unwired: 1 in, 1 out]
            n106 = global read "Global_flags.vi" "Open / Close COM?"() -> (w507:bool)
            n107 = global read "Global_flags.vi" "Calib Data?"() -> (w508:bool)
            n108 = And(x=w508, y=w507) -> (x .and. y?=w506:bool)
            n109 = case shown="True" w506 {
              tunnel: w512 -> [w519 w528]
              tunnel: [w519 w527] -> w511
              tunnel: w510 -> [w518 w526]
              tunnel: [w518 w525] -> w509
              frame False {
                # "Solo se puede CONFIRM SLOPE si el COM esta abierto y estamos en CALIBRACION"
                n110 = Concatenate Strings("Para CONFIRMAR SLOPE::::::" ("message"), "\r\n", "Debe ABRIR Puerto COM o Start Calibracion (ADC) Primero !!!" ("string")) -> (w517:string)
                n111 = One Button Dialog(message=w517, button name ("OK")="Aceptar") -> ()  [unwired: 1 out]
              }
              frame True {
                w530 = FSM_States."Confirm Slope"  # Next State
                # "Solo se puede CONFIRM SLOPE si el COM esta abierto y estamos en CALIBRACION"
                n112 = Concatenate Strings("FIN de la Calibracion" ("string"), "\r\n", "MODO de Lectura RE-establecido" ("string")) -> (w523:string)
                n113 = Bundle By Name(cluster=T1 {"Consumer State"=enum."Open COM Port", "User Msg"="", "error in (no error)"={"status"=FALSE, "code"=0, "source"=""}, "User Msg 2"=""} ("Global Message"), "Consumer State"=w530, "User Msg"="OK SLOPE Confirmado !!", "User Msg 2"=w523) -> (w524:T1)
                n114 = Enqueue Element At Opposite End(queue=w528, element=w524, error in (no error)=w526) -> (queue out=w527:refnum<queue>, error out=w525:errorcluster)  [unwired: 1 in, 1 out]
              }
            }
          }
          event "Exit": Value Change {
            # "Esta abierto el puerto COM???"
            n115 = event-data() -> ()  [unwired: 1 in, 1 out]
            n116 = global read "Global_flags.vi" "Open / Close COM?"() -> (w533:bool)
            n117 = case shown="True" w533 {
              tunnel: w537 -> [w543 w547]
              tunnel: [w542 w547] -> w536
              tunnel: w535 -> [w541 w546]
              tunnel: [w540 w546] -> w534
              tunnel: [TRUE FALSE] -> w532
              frame False {
                w544 = FSM_States."Exit App"  # Next State
                # "Solo se puede EXIT si el puerto COM esta cerrado"
                n118 = Bundle By Name(cluster=T1 {"Consumer State"=enum."Open COM Port", "User Msg"="", "error in (no error)"={"status"=FALSE, "code"=0, "source"=""}, "User Msg 2"=""} ("Global Message"), "Consumer State"=w544) -> (w539:T1)
                n119 = Enqueue Element At Opposite End(queue=w543, element=w539, error in (no error)=w541) -> (queue out=w542:refnum<queue>, error out=w540:errorcluster)  [unwired: 1 in, 1 out]
              }
              frame True {
              }
            }
          }
          event Panel Close? {
            # "Cerra el Panel Frontal"
            n120 = event-data() -> ()  [unwired: 1 in, 2 out]
            n121 = Two Button Dialog(message="Esta Seguro de salir?", 1:"Cancelar" ("F button name (\"Cancel\")"), 2:"Aceptar" ("T button name (\"OK\")")) -> (T button?=w553:bool)
            n122 = Not(x=w553) -> (.not. x?=w552:bool)
            n123 = event-data("Discard?"=w552) -> ()  [unwired: 1 in, 1 out]
          }
        }
        n124 = Or(x=w256, y=w257) -> (x .or. y?=w255:bool)
        n125 = call "Error Handler.vi"("error in (no error)"=w256, "Queue in"=w260) -> ("error out"=w258:errorcluster, "Queue out"=w259:refnum<queue>)  [unwired: 8 in]
      }
      n126 = while {
        tunnel: w12 -> [w39]
        shift-right: [w34] -> _
        shift-left: refnum<class "Modbus Master.lvclass"> refnum ("serial master instance") -> [w33]
        shift-right: [w30] -> _
        shift-left: errorcluster {"status"=FALSE, "code"=0, "source"=""} ("error out") -> [w32]
        shift-right: [w27] -> w3
        shift-left: w11 -> [w38]
        shift-right: [w22] -> _
        shift-left: refnum<file> refnum ("refnum out") -> [w20]
        shift-right: [w21] -> _
        shift-left: errorcluster {"status"=FALSE, "code"=0, "source"=""} ("error out") -> [w19]
        stop <- w26 stop-if-true
        # "Bucle de Consumo y de Adquisicion"
        n127 = Dequeue Element(queue=w39, error in (no error)=w38) -> (queue out=w31:refnum<queue>, element=w37:T1, error out=w29:errorcluster)  [unwired: 1 in, 1 out]
        n128 = Unbundle By Name(w37) -> ("User Msg 2"=w23:string, "User Msg"=w35:string, "Consumer State"=w36:T2, "error in (no error)"=w25:errorcluster)
        n129 = case shown="\"Calibrate sensor\"" w36 {
          tunnel: w35 -> [_ w78 _ w117 w128 w139 w153 w170 w187 _ _ _ w243]
          tunnel: [w68 w74 w105 w122 w132 w142 w158 w173 _ w202 w211 w235 w248] -> w34
          tunnel: [w67 w73 w104 w118 w129 w140 w154 w171 w188 w196 w210 w231 w244] -> w30
          tunnel: w33 -> [w68 _ w103 w123 w133 w143 w159 w174 w189 w202 w211 w236 w250]
          tunnel: w32 -> [w67 _ w102 w121 w131 w141 w157 w172 w190 w199 w210 w234 w249]
          tunnel: [_ _ _ _ _ _ _ _ _ TRUE _ _ _] -> w24
          tunnel: w25 -> [_ _ _ _ _ _ _ _ _ w200 _ _ _]
          tunnel: w23 -> [_ _ _ _ _ _ w152 w167 _ _ _ _ w246]
          tunnel: [w41 w72 w91 w116 w127 w138 w149 w166 w184 w195 w204 w214 w242] -> w22
          tunnel: [w40 w71 w90 w115 w126 w137 w148 w165 w183 w193 w203 w213 w241] -> w21
          tunnel: w20 -> [_ w72 w91 w116 w127 w138 w149 w166 w184 w195 w204 w216 w242]
          tunnel: w19 -> [_ w71 w90 w115 w126 w137 w148 w165 w183 w194 w203 w215 w241]
          frame "Initialize", Default {
            w58 = T3."Enabled" ("Disabled")
            w63 = sgl 0.0 ("Measurement [%  ; mg/L]:")
            # "Comma"
            # "Y"
            # "AGREGAR MEMBRETE"
            # "X"
            # "CREAR REPORTE DE CALIBRACION"
            # "IDLE STATE  : Init alll variables"
            n130 = local write "Measurement [%  ; mg/L]:"(w63) -> ()
            n131 = local write "Temperature [°C]:"(w63) -> ()
            n132 = local write "Current Out Val :"(w63) -> ()
            n133 = local write "Warning :"("") -> ()
            n134 = property on="Measurement [%  ; mg/L]:" class="DigNum (strict)"(error in=errorcluster {"status"=FALSE, "code"=0, "source"=""} ("error in (no error)"), "DisabledEnum"=w58) -> (error out=w59:errorcluster)  [unwired: 1 in, 1 out]
            n135 = call "Create Data File.vi"("error in"=errorcluster {"status"=FALSE, "code"=0, "source"=""}, "UUT"="DO_Sensor") -> ("error out"=w44:errorcluster, "refnum out"=w45:refnum<file>)  [unwired: 8 in]
            n136 = local write "Consumer Shutdown?"(FALSE ("Consumer Shutdown?")) -> ()
            n137 = property on="Consumer Shutdown?" class="Bool (strict)"("Visible"=FALSE) -> ()  [unwired: 2 in, 2 out]
            n138 = property on="Adquire / Stop" class="Bool"("Strings [4]"=string[] ["GO"]) -> ()  [unwired: 2 in, 2 out]
            n139 = property on="Temperature [°C]:" class="DigNum (strict)"(error in=w59, "DisabledEnum"=w58) -> (error out=w60:errorcluster)  [unwired: 1 in, 1 out]
            n140 = property on="Current Out Val :" class="DigNum (strict)"(error in=w60, "DisabledEnum"=w58) -> (error out=w61:errorcluster)  [unwired: 1 in, 1 out]
            n141 = property on="Start Calib" class="Bool"("DisabledEnum"=T3."Enabled" ("Disabled")) -> ()  [unwired: 2 in, 2 out]
            n142 = property on="Start Calib" class="Bool"("Strings [4]"=string[] ["Start"]) -> ()  [unwired: 2 in, 2 out]
            n143 = Concatenate Strings("HORA/TIEMPO" ("string"), "," ("string"), "MUESTRA ADC" ("string"), "\r\n") -> (w43:string)
            n144 = global write "Global_flags.vi" "Adquire /Stop DATA?"(FALSE ("Adquire /Stop DATA?")) -> ()
            n145 = global write "Global_flags.vi" "Open / Close COM?"(FALSE ("Open / Close COM?")) -> ()
            n146 = global write "Global_flags.vi" "Calib Data?"(FALSE ("Calib Data?")) -> ()
            n147 = property on="Warning :" class="Str"(error in=w61, "DisabledEnum"=w58) -> ()  [unwired: 1 in, 2 out]
            n148 = property on="Open/Close COM" class="Bool"("Strings [4]"=string[] ["OpenCOM"]) -> ()  [unwired: 2 in, 2 out]
            n149 = Write to Text File(file (use dialog)=w45, text=w43, error in=w44) -> (refnum out=w41:refnum<file>, error out=w40:errorcluster)  [unwired: 1 in, 1 out]
            n150 = property on="Tiempo Actual" class="Str"("Visible"=FALSE) -> ()  [unwired: 2 in, 2 out]
            n151 = property on="ADC" class="DigNum (strict)"("DisabledEnum"=T3."Disabled and Grayed Out" ("Disabled")) -> ()  [unwired: 2 in, 2 out]
          }
          frame "Open COM Port" {
            w82 = u16 0 items=["None", "Odd", "Even"] ("parity (Even)")
            w83 = enum16{"RTU", "ASCII"}."RTU"  # serial type
            # "Configurar puerto COM Modbus"
            # "No errors"
            # "No check  bit"
            # "Abiri la instancia de Maestro Modbus segun los controles : \n\"Address\", \"COM\", \"BaudRate,...."
            n152 = call-poly <vilib>:"Create Master Instance.vi"("serial type"=w83, "parity (Even)"=w82, "unit ID"="Address", "error in (no error)"=errorcluster {"status"=FALSE, "code"=0, "source"=""}, "baud rate (9600)"="BaudRate (9600)", "VISA resource name"="COM") -> ("error out"=w73:errorcluster, "serial master instance"=w74:refnum<class "Modbus Master.lvclass">)  [unwired: 4 in]
            n153 = case shown="No Error" w73 {
              tunnel: [string[] ["CloseCOM"] ("Strings [4]") string[] ["OpenCOM"] ("Strings [4]")] -> w79
              tunnel: [TRUE ("Open / Close COM?") FALSE ("Open / Close COM?")] -> w80
              tunnel: w78 -> [w84 _]
              frame No Error {
                # "If open sucess ..."
                n154 = One Button Dialog(message=w84, button name ("OK")="Aceptar") -> ()  [unwired: 1 out]
              }
              frame Error {
              }
            }
            n155 = global write "Global_flags.vi" "Open / Close COM?"(w80) -> ()
            n156 = property on="Open/Close COM" class="Bool"("Strings [4]"=w79) -> ()  [unwired: 2 in, 2 out]
          }
          frame "Adquire Data" {
            # "Resolucion: ????????"
            # "Resolucion: 0.1 °C"
            # "Resolucion: 0.01 mg/L"
            # "No calibrar si solo se ADQUIERE!!"
            # "Hasta el registro del MEASUREMENT MODE (0x0008)"
            # "Desde el registro MEASUREMENTS[ CD AB] (0x0001)"
            # "Adquirir la Data del sensor y mostrar en GUI pantalla"
            n157 = call-dynamic "Read Holding Registers.vi"("error in (no error)"=w102, "number of holding registers"=u16 8, "starting address"=u16 1, "Modbus master in"=w103) -> ("error out"=w104:errorcluster, "register values"=w100:u16[], "Modbus master out"=w105:refnum<class "Modbus Master.lvclass">)  [unwired: 5 in]
            n158 = call "Return Reg Values.vi"("Register Values"=w100) -> ("Measure Mode"=w94:u16, "Current Output value"=→"Current Out Val :":sgl, "Temperature Measurement"=→"Temperature [°C]:":sgl, "Measurements"=→"Measurement [%  ; mg/L]:":sgl, "Warning"=→"Warning :":string)  [unwired: 6 in]
            n159 = case shown="No Error" w104 {
              tunnel: [TRUE FALSE] -> w106
              tunnel: [string[] ["STOP"] ("Strings [4]") string[] ["GO"] ("Strings [4]")] -> w101
              frame No Error {
                # "Start Adq ..."
              }
              frame Error {
                # "Could not Adq Data"
              }
            }
            n160 = case shown="1" w94 {
              tunnel: ["%#.2f %" "%#.2f mg/L"] -> w93
              frame 0, Default {
                # "00: %  ; 01: mg/L"
              }
              frame 1 {
                # "00: %  ; 01: mg/L"
              }
            }
            n161 = property on="Tiempo Actual" class="Str"("Visible"=FALSE) -> ()  [unwired: 2 in, 2 out]
            n162 = property on="Measurement [%  ; mg/L]:" class="DigNum (strict)"("FormatString"=w93) -> ()  [unwired: 2 in, 2 out]
            n163 = global write "Global_flags.vi" "Adquire /Stop DATA?"(w106) -> ()
            n164 = global write "Global_flags.vi" "Calib Data?"(FALSE ("Calib Data?")) -> ()
            n165 = property on="Adquire / Stop" class="Bool"("Strings [4]"=w101) -> ()  [unwired: 2 in, 2 out]
          }
          frame "Set Address" {
            # "Resgistro DEVICE ADDRESS (0x0019)"
            # "Default Value : 1"
            # "Cambiar la direccion Modbus SLAVE ID del dispositivo"
            n166 = call-dynamic "Write Single Holding Register.vi"("error in (no error)"=w121, "holding register value"="Addr Set", "address"=u16 25, "Modbus master in"=w123) -> ("error out"=w118:errorcluster, "Modbus master out"=w122:refnum<class "Modbus Master.lvclass">)  [unwired: 6 in]
            n167 = case shown="No Error" w118 {
              tunnel: w117 -> [w125 _]
              frame No Error {
                n168 = One Button Dialog(message=w125, button name ("OK")="Aceptar") -> ()  [unwired: 1 out]
              }
              frame Error {
              }
            }
          }
          frame "Set BaudRate" {
            # "Resgistro BAUDRATE (0x001A)"
            # "Default Value : 9600"
            # "Change Baudrate  \nCAUTION : The device may stop working"
            n169 = call-dynamic "Write Single Holding Register.vi"("error in (no error)"=w131, "holding register value"="BaudRate (9600)", "address"=u16 26, "Modbus master in"=w133) -> ("error out"=w129:errorcluster, "Modbus master out"=w132:refnum<class "Modbus Master.lvclass">)  [unwired: 6 in]
            n170 = case shown="No Error" w129 {
              tunnel: w128 -> [w135 _]
              frame No Error {
                n171 = One Button Dialog(message=w135, button name ("OK")="Aceptar") -> ()  [unwired: 1 out]
              }
              frame Error {
              }
            }
          }
          frame "Restore Factory" {
            # "Resgistro RESTORE DEFAULT (0x001B)"
            # "Restore Default CMD : Addr =1, BaudRate=9600"
            # "Restablecer el sensor a valores de fabrica"
            n172 = call-dynamic "Write Single Holding Register.vi"("error in (no error)"=w141, "holding register value"=u16 255, "address"=u16 27, "Modbus master in"=w143) -> ("error out"=w140:errorcluster, "Modbus master out"=w142:refnum<class "Modbus Master.lvclass">)  [unwired: 6 in]
            n173 = case shown="No Error" w140 {
              tunnel: w139 -> [w147 _]
              frame No Error {
                n174 = One Button Dialog(message=w147, button name ("OK")="Aceptar") -> ()  [unwired: 1 out]
              }
              frame Error {
              }
            }
          }
          frame "Confirm Zero" {
            # "RE-Establecer el MODO de LECTURA"
            # "SALIR DEL MODO CALIBRACION"
            # "Resgistro ZERO CALIBRATION (0x003E)"
            # "Comando de Confirmacion de ZERO"
            # "Confirmacion del PUNTO ZERO"
            n175 = call-dynamic "Write Single Holding Register.vi"("error in (no error)"=w157, "holding register value"=u16 255, "address"=u16 62, "Modbus master in"=w159) -> ("error out"=w154:errorcluster, "Modbus master out"=w158:refnum<class "Modbus Master.lvclass">)  [unwired: 6 in]
            n176 = case shown="No Error" w154 {
              tunnel: w153 -> [w161 _]
              tunnel: w152 -> [w160 _]
              frame No Error {
                n177 = flat-sequence {
                  tunnel: w161 -> [w163]
                  tunnel: w160 -> [w164]
                  frame #0 {
                    n178 = One Button Dialog(message=w163, button name ("OK")="Aceptar") -> ()  [unwired: 1 out]
                  }
                  frame #1 {
                    n179 = One Button Dialog(message=w164) -> ()  [unwired: 1 in, 1 out]
                  }
                }
              }
              frame Error {
              }
            }
            n180 = global write "Global_flags.vi" "Adquire /Stop DATA?"(TRUE ("Adquire /Stop DATA?")) -> ()
            n181 = global write "Global_flags.vi" "Calib Data?"(FALSE ("Calib Data?")) -> ()
          }
          frame "Confirm Slope" {
            # "RE-Establecer el MODO de LECTURA"
            # "Resgistro SLOPE CALIBRATION (0x003F)"
            # "SALIR DEL MODO CALIBRACION"
            # "Confirmacion del PUNTO SLOPE"
            n182 = call-dynamic "Write Single Holding Register.vi"("error in (no error)"=w172, "holding register value"=u16 255, "address"=u16 63, "Modbus master in"=w174) -> ("error out"=w171:errorcluster, "Modbus master out"=w173:refnum<class "Modbus Master.lvclass">)  [unwired: 6 in]
            n183 = case shown="No Error" w171 {
              tunnel: w170 -> [w178 _]
              tunnel: w167 -> [w177 _]
              frame No Error {
                n184 = flat-sequence {
                  tunnel: w178 -> [w179]
                  tunnel: w177 -> [w182]
                  frame #0 {
                    n185 = One Button Dialog(message=w179, button name ("OK")="Aceptar") -> ()  [unwired: 1 out]
                  }
                  frame #1 {
                    n186 = One Button Dialog(message=w182, button name ("OK")="Aceptar") -> ()  [unwired: 1 out]
                  }
                }
              }
              frame Error {
              }
            }
            n187 = global write "Global_flags.vi" "Adquire /Stop DATA?"(TRUE ("Adquire /Stop DATA?")) -> ()
            n188 = global write "Global_flags.vi" "Calib Data?"(FALSE ("Calib Data?")) -> ()
          }
          frame "Close COM Port" {
            # "CERRAR EL PUERTO COM del Modbus"
            n189 = call-dynamic "Close.vi"("error in (no error)"=w190, "Modbus master in"=w189) -> ("error out"=w188:errorcluster)  [unwired: 9 in]
            n190 = case shown="No Error" w188 {
              tunnel: w187 -> [w192 _]
              frame No Error {
                n191 = One Button Dialog(message=w192, button name ("OK")="Aceptar") -> ()  [unwired: 1 out]
              }
              frame Error {
              }
            }
            n192 = global write "Global_flags.vi" "Open / Close COM?"(FALSE ("Open / Close COM?")) -> ()
            n193 = property on="Open/Close COM" class="Bool"("Strings [4]"=string[] ["OpenCOM"]) -> ()  [unwired: 2 in, 2 out]
          }
          frame "Exit App" {
            w197 = T4 1 items=["no dialog", "OK message", "continue or stop message", "OK message + warnings", "continue/stop + warnings"] ("type of dialog (OK msg:1)")
            # "Data Comunication errors are reported here"
            # "Releases the queue"
            # "Releases queue and EXIT App"
            n194 = Merge Errors(w200, w199) -> (w198:errorcluster)
            n195 = call <vilib>:"Simple Error Handler.vi"("type of dialog (OK msg:1)"=w197, "error in (no error)"=w198) -> ("error out"=w196:errorcluster)  [unwired: 3 in, 4 out]
            n196 = Close File(refnum=w195, error in=w194) -> (error out=w193:errorcluster)  [unwired: 1 out]
          }
          frame "Stop Data" {
            w207 = sgl 0.0 ("Measurement [%  ; mg/L]:")
            # "DEJAR DE ADQUIRIR"
            # "DETENER LA TOMA DE MUESTRAS"
            n197 = property on="Adquire / Stop" class="Bool"("Strings [4]"=string[] ["GO"]) -> ()  [unwired: 2 in, 2 out]
            n198 = local write "ADC"(u16 0 ("ADC")) -> ()
            n199 = global write "Global_flags.vi" "Adquire /Stop DATA?"(FALSE ("Adquire /Stop DATA?")) -> ()
            n200 = local write "Measurement [%  ; mg/L]:"(w207) -> ()
            n201 = local write "Warning :"("") -> ()
            n202 = local write "Temperature [°C]:"(w207) -> ()
            n203 = local write "Current Out Val :"(w207) -> ()
          }
          frame "Calibrate sensor" {
            # "ESCRIBIR EN REPORTE"
            # "Dato ADC"
            # "comma"
            # "Hora:Minuto:Segundo"
            # "# de Registros a leer"
            # "Resgistro ADC (0x0066)"
            # "No se debe leer sensor si aun se calibra"
            # "Valor ADC"
            # "Leer el valor ADC para poder calibrar"
            n204 = Format Date/Time String(time format string (%c)="%H : %M : %S ") -> (date/time string=→"Tiempo Actual":string)  [unwired: 2 in]
            n205 = call-dynamic "Read Holding Registers.vi"("error in (no error)"=w234, "number of holding registers"=u16 1, "starting address"=u16 102, "Modbus master in"=w236) -> ("error out"=w231:errorcluster, "register values"=w228:u16[], "Modbus master out"=w235:refnum<class "Modbus Master.lvclass">)  [unwired: 5 in]
            n206 = Format Date/Time String(time format string (%c)="%H:%M%S") -> (date/time string=w222:string)  [unwired: 2 in]
            n207 = Index Array(array=w228, index=0) -> (element=w212:u16)
            "ADC" <- w212
            n208 = Format Into String(format string="%04d", w212) -> (resulting string=w220:string)  [unwired: 2 in, 1 out]
            n209 = case shown="No Error" w231 {
              tunnel: [TRUE FALSE] -> w230
              tunnel: [TRUE ("Visible") FALSE ("Visible")] -> w224
              frame No Error {
              }
              frame Error {
              }
            }
            n210 = Concatenate Strings(w222, "," ("string"), w220, "\r\n") -> (w217:string)
            n211 = global write "Global_flags.vi" "Adquire /Stop DATA?"(FALSE ("Adquire /Stop DATA?")) -> ()
            n212 = global write "Global_flags.vi" "Calib Data?"(w230) -> ()
            n213 = Write to Text File(file (use dialog)=w216, text=w217, error in=w215) -> (refnum out=w214:refnum<file>, error out=w213:errorcluster)  [unwired: 1 in, 1 out]
            n214 = property on="Tiempo Actual" class="Str"("Visible"=w224) -> ()  [unwired: 2 in, 2 out]
          }
          frame "Set Measure Mode" {
            # "Resgistro MEASUREMENT MODE (0x0008)"
            # "Cambiar la direccion Modbus SLAVE ID del dispositivo"
            n215 = case shown="\"%\"" w246 {
              tunnel: [u16 1 ("holding register value") u16 0 ("holding register value")] -> w245
              frame "mg/L", Default {
              }
              frame "%" {
                # "[%]  o [mg/L]"
              }
            }
            n216 = call-dynamic "Write Single Holding Register.vi"("error in (no error)"=w249, "holding register value"=w245, "address"=u16 8, "Modbus master in"=w250) -> ("error out"=w244:errorcluster, "Modbus master out"=w248:refnum<class "Modbus Master.lvclass">)  [unwired: 6 in]
            n217 = case shown="No Error" w244 {
              tunnel: w243 -> [w252 _]
              frame No Error {
                n218 = One Button Dialog(message=w252, button name ("OK")="Aceptar") -> ()  [unwired: 1 out]
              }
              frame Error {
              }
            }
          }
        }
        "Consumer Shutdown?" <- w24
        n219 = Merge Errors(w29, w30, w21) -> (w28:errorcluster)
        n220 = call "Error Handler.vi"("error in (no error)"=w28, "Queue in"=w31) -> ("error out"=w27:errorcluster)  [unwired: 8 in, 1 out]
        n221 = Or(x=w27, y=w24) -> (x .or. y?=w26:bool)
      }
      n222 = Release Queue(queue=w8, error in (no error)=w7) -> (error out=w4:errorcluster)  [unwired: 1 in, 2 out]
      n223 = Merge Errors(w4, w3) -> (w6:errorcluster)
      n224 = call <vilib>:"Simple Error Handler.vi"("type of dialog (OK msg:1)"=w5, "error in (no error)"=w6) -> ()  [unwired: 3 in, 5 out]
    }
    frame #1 {
      n225 = disable-structure shown="RUN_TIME_ENGINE==False, Default" {
        disable-tunnel: [TRUE FALSE] -> w556
        frame condition #0 {
        }
        frame condition #1 (active) {
        }
      }
      n226 = Quit LabVIEW(quit? (T)=w556) -> ()
    }
  }
